vi "Format Time for RPI.vi"() -> (2 "is date valid?":bool, 3 "date/time string":string)   [LabVIEW 2025]
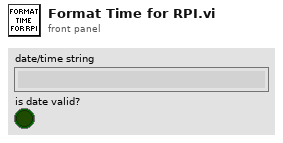
[diagram p1: front panel]
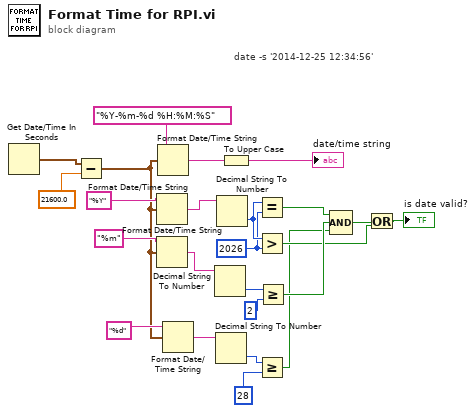
[diagram p0: block diagram]
diagram:
  w19 = 2026 ("y")
  # "date -s '2014-12-25 12:34:56'"
  n1 = Get Date/Time In Seconds() -> (seconds since 1Jan1904=w2:timestamp)
  n2 = Subtract(x=w2, y=21600.0) -> (x-y=w1:timestamp)
  n3 = Format Date/Time String(time format string (%c)="%Y", seconds (now)=w1) -> (date/time string=w21:string)  [unwired: 1 in]
  n4 = Format Date/Time String(time format string (%c)="%m", seconds (now)=w1) -> (date/time string=w18:string)  [unwired: 1 in]
  n5 = Format Date/Time String(time format string (%c)="%Y-%m-%d %H:%M:%S", seconds (now)=w1) -> (date/time string=w10:string)  [unwired: 1 in]
  n6 = Format Date/Time String(time format string (%c)="%d", seconds (now)=w1) -> (date/time string=w8:string)  [unwired: 1 in]
  n7 = Decimal String To Number(string=w18) -> (number=w17:i32)  [unwired: 2 in, 1 out]
  n8 = Decimal String To Number(string=w8) -> (number=w6:i32)  [unwired: 2 in, 1 out]
  n9 = Decimal String To Number(string=w21) -> (number=w20:i32)  [unwired: 2 in, 1 out]
  n10 = To Upper Case(1:w10) -> (0:→"date/time string":string)
  n11 = Equal?(x=w20, y=w19) -> (x = y?=w15:bool)
  n12 = Greater?(x=w20, y=w19) -> (0:w12:bool)
  n13 = Greater Or Equal?(x=w6, y=28) -> (x >= y?=w4:bool)
  n14 = Greater Or Equal?(x=w17, y=2) -> (x >= y?=w14:bool)
  n15 = Compound Arithmetic op=AND(w15, w14, w4) -> (w13:bool)
  n16 = Or(x=w13, y=w12) -> (x .or. y?=→"is date valid?":bool)
